vi "Regular Waves (Modded by Matt).vi"(0 "Run":bool, 1 "Wave Period":dbl(slide)=1.0 min=0.5 max=5.0 step=0.01 scale=0.5..5.0 scale format="%.1f", 2 "Wave Height":dbl(slide)=0.1 min=0.0 step=0.001 scale=0.0..0.15606733627984637 scale format="%.3f") -> ()   [LabVIEW 2012]
uses:
  <vilib>/Daq/Ai.llb/AI Read (scaled array).vi
  <vilib>/Daq/ao.llb/AO Write (scaled array).vi
  <vilib>/Daq/ao.llb/AO Write One Update (scaled array).vi
  <vilib>/Analysis/NI_AALBase.lvlib
  <vilib>/Analysis/1siggen.llb/Ramp Pattern by Samples.vi
panel:
  out "Waveform Chart":dbl[][](graph)
  in  "Measure Waves":bool
  in  "Settings":bool
  in  "Power":bool
  out "Buffer Size":i32=4000
  # "Regular Wave Generator"
  # "s"
  # "m"
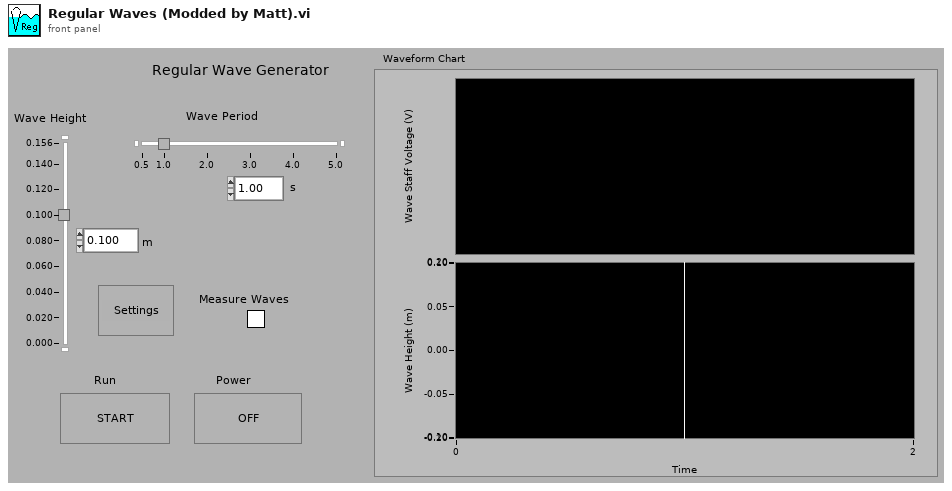
[diagram p1: front panel]
types:
  T1 = cluster{"Output Device":i16, "Output Channel":string, "Sampling Rate (Hz)":dbl, "Input Device":i16, "Input Channel":string, "Input Offset (V)":dbl, "Input Calibration (m/V)":dbl, "Stroke Calibration (V/m)":dbl, "Paddle Height (m)":dbl, "Water Depth (m)":dbl, "Min Period":dbl, "Max Period":dbl, "Max 1/2 Piston Stroke":dbl, "Max H/L":dbl, "Max H/d":dbl}
  T2 = cluster{"Period":dbl, "Wave Height":dbl, "Phase Angle (rad)":dbl}
  T3 = cluster{"Sampling Rate":i32, "Water Depth":dbl, "Paddle Height":dbl}
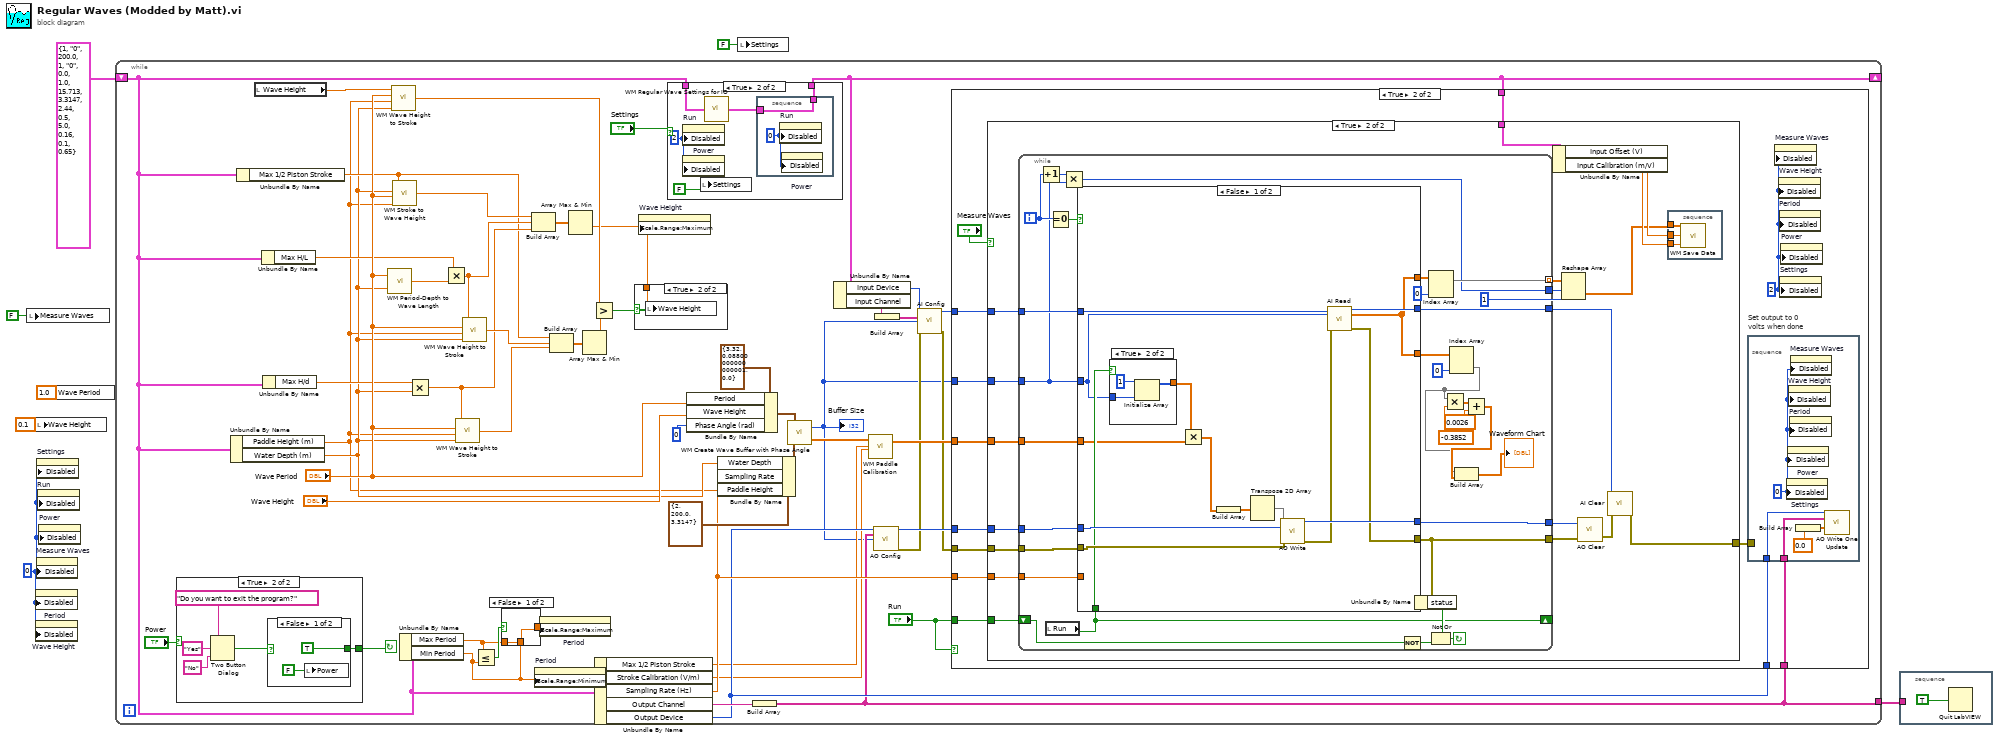
[diagram p0: block diagram]
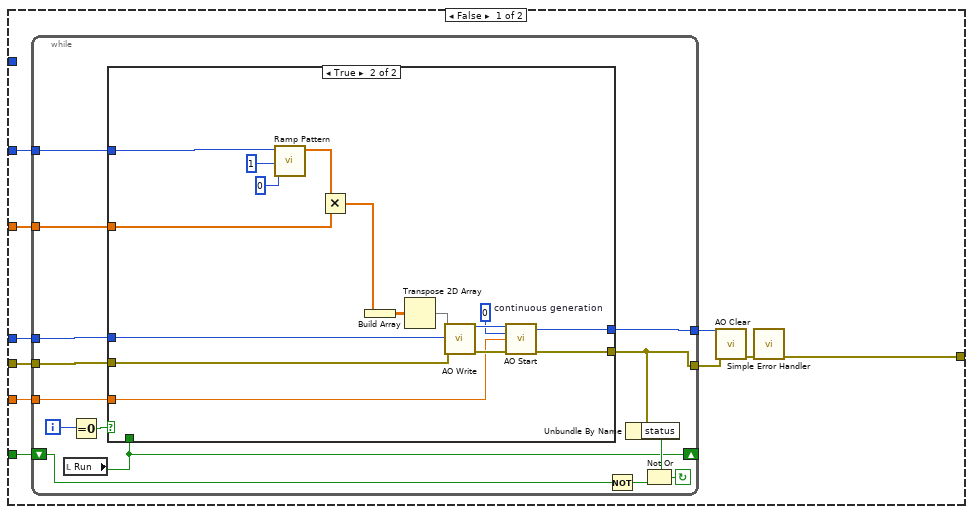
[diagram p3: hidden frame]
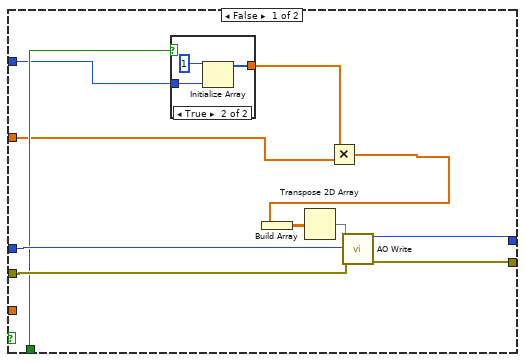
[diagram p4: hidden frame]
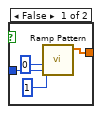
[diagram p5: hidden frame]
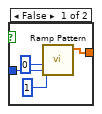
[diagram p6: hidden frame]
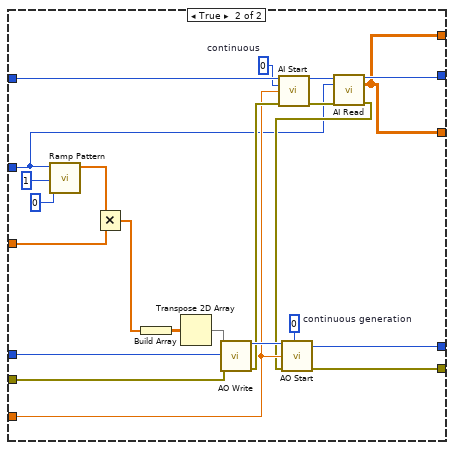
[diagram p7: hidden frame]
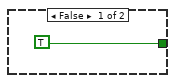
[diagram p9: hidden frame]
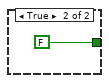
[diagram p10: hidden frame]
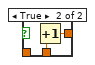
[diagram p11: hidden frame]
diagram:
  w2 = u8 0 ("Write Attribute")
  n1 = local write "Measure Waves"(FALSE ("Measure Waves")) -> ()
  n2 = local write "Wave Height"(0.1 ("Wave Height")) -> ()
  n3 = property on="Period" class="Slide (strict)"("Disabled"=w2) -> ()  [unwired: 2 in, 2 out]
  n4 = property on="Wave Height" class="Slide (strict)"("Disabled"=w2) -> ()  [unwired: 2 in, 2 out]
  n5 = property on="Measure Waves" class="Bool (strict)"("Disabled"=w2) -> ()  [unwired: 2 in, 2 out]
  n6 = property on="Settings" class="Bool (strict)"("Disabled"=w2) -> ()  [unwired: 2 in, 2 out]
  n7 = property on="Run" class="Bool (strict)"("Disabled"=w2) -> ()  [unwired: 2 in, 2 out]
  n8 = property on="Power" class="Bool (strict)"("Disabled"=w2) -> ()  [unwired: 2 in, 2 out]
  n9 = local write "Wave Period"(1.0 ("Period")) -> ()
  n10 = while {
    shift-left: T1 {"Output Device"=1, "Output Channel"="0", "Sampling Rate (Hz)"=200.0, "Input Device"=1, "Input Channel"="0", "Input Offset (V)"=0.0, "Input Calibration (m/V)"=1.0, "Stroke Calibration (V/m)"=15.713, "Paddle Height (m)"=3.3147, "Water Depth (m)"=2.44, "Min Period"=0.5, "Max Period"=5.0, "Max 1/2 Piston Stroke"=0.16, "Max H/L"=0.1, "Max H/d"=0.65} ("Settings") -> [w19]
    shift-right: [w8] -> _
    tunnel: [w27] -> w7
    stop <- w43 continue-if-true
    n11 = case shown="True" "Power" {
      tunnel: [TRUE w240] -> w43
      frame False {
      }
      frame True {
        n12 = Two Button Dialog(message="Do you want to exit the program?", 1:"No" ("F button name (\"Cancel\")"), 2:"Yes" ("T button name (\"OK\")")) -> (T button?=w241:bool)
        n13 = case shown="False" w241 {
          tunnel: [TRUE FALSE] -> w240
          frame False {
            n14 = local write "Power"(FALSE ("Power")) -> ()
          }
          frame True {
          }
        }
      }
    }
    n15 = Unbundle By Name(w19) -> ("Paddle Height (m)"=w22:dbl, "Water Depth (m)"=w23:dbl)
    n16 = Unbundle By Name(w19) -> ("Max 1/2 Piston Stroke"=w26:dbl)
    n17 = local read "Wave Height"() -> (w46:dbl)
    n18 = Unbundle By Name(w19) -> ("Max H/L"=w25:dbl)
    n19 = Unbundle By Name(w19) -> ("Max H/d"=w24:dbl)
    n20 = call "WM Period-Depth to Wave Length.vi"("Water Depth"=w23, "Period"="Wave Period") -> ("WaveLength"=w34:dbl)
    n21 = call "WM Wave Height to Stroke.vi"("Water Depth (m)"=w23, "Flap Height (m)"=w22, "Wave Period (s)"="Wave Period", "Wave Height (m)"=w46) -> ("Flap Amplitude (from x=0) (m)"=w55:dbl)
    n22 = call "WM Stroke to Wave Height.vi"("Paddle Height (m)"=w22, "Wave Period (s)"="Wave Period", "Water Depth (m)"=w23, "Flap Amplitude from x=0 (m)"=w26) -> ("Wave Height (m)"=w50:dbl)
    n23 = Unbundle By Name(w19) -> ("Max Period"=w18:dbl, "Min Period"=w17:dbl)
    n24 = Multiply(x=w24, y=w23) -> (x*y=w33:dbl)
    n25 = Multiply(x=w25, y=w34) -> (x*y=w51:dbl)
    n26 = call "WM Wave Height to Stroke.vi"("Water Depth (m)"=w23, "Flap Height (m)"=w22, "Wave Period (s)"="Wave Period", "Wave Height (m)"=w33) -> ("Flap Amplitude (from x=0) (m)"=w49:dbl)
    n27 = call "WM Wave Height to Stroke.vi"("Water Depth (m)"=w23, "Flap Height (m)"=w22, "Wave Period (s)"="Wave Period", "Wave Height (m)"=w51) -> ("Flap Amplitude (from x=0) (m)"=w48:dbl)
    n28 = Less Or Equal?(x=w18, y=w17) -> (x <= y?=w56:bool)
    n29 = case shown="False" w56 {
      tunnel: w17 -> [_ w250]
      tunnel: [w248 w249] -> w45
      tunnel: w18 -> [w248 _]
      frame False {
      }
      frame True {
        n30 = Increment(x=w250) -> (x+1=w249:dbl)
      }
    }
    n31 = Build Array(w50, w51, w33) -> (w54:dbl[])
    n32 = property on="Period" class="Slide (strict)"("Scale.Range:Minimum"=w17) -> ()  [unwired: 2 in, 2 out]
    n33 = property on="Period" class="Slide (strict)"("Scale.Range:Maximum"=w45) -> ()  [unwired: 2 in, 2 out]
    n34 = Build Array(w26, w48, w49) -> (w53:dbl[])
    n35 = Array Max & Min(array=w54) -> (min value=w47:dbl)  [unwired: 3 out]
    n36 = Array Max & Min(array=w53) -> (min value=w52:dbl)  [unwired: 3 out]
    n37 = Greater?(x=w55, y=w52) -> (0:w57:bool)
    n38 = Unbundle By Name(w19) -> ("Max 1/2 Piston Stroke"=w21:dbl, "Stroke Calibration (V/m)"=w20:dbl, "Sampling Rate (Hz)"=w30:dbl, "Output Channel"=w29:string, "Output Device"=w28:i16)
    n39 = case shown="True" w57 {
      tunnel: w47 -> [_ w251]
      frame False {
      }
      frame True {
        n40 = local write "Wave Height"(w251) -> ()
      }
    }
    n41 = property on="Wave Height" class="Slide (strict)"("Scale.Range:Maximum"=w47) -> ()  [unwired: 2 in, 2 out]
    n42 = case shown="True" "Settings" {
      tunnel: w19 -> [w231 w236]
      tunnel: [w231 w234] -> w8
      frame False {
      }
      frame True {
        w232 = u8 2 ("Write Attribute")
        n43 = property on="Run" class="Bool (strict)"("Disabled"=w232) -> ()  [unwired: 2 in, 2 out]
        n44 = property on="Power" class="Bool (strict)"("Disabled"=w232) -> ()  [unwired: 2 in, 2 out]
        n45 = local write "Settings"(FALSE ("Settings")) -> ()
        n46 = call "WM Regular Wave Settings for IO.vi"("Settings"=w236) -> ("Settings Output"=w235:T1)
        n47 = stacked-sequence {
          tunnel: w235 -> [w238]
          tunnel: [w238] -> w234
          frame #0 {
            w237 = u8 0 ("Write Attribute")
            n48 = property on="Run" class="Bool (strict)"("Disabled"=w237) -> ()  [unwired: 2 in, 2 out]
            n49 = property on="Power" class="Bool (strict)"("Disabled"=w237) -> ()  [unwired: 2 in, 2 out]
          }
        }
      }
    }
    n50 = Bundle By Name(cluster=T2 {"Period"=3.32, "Wave Height"=0.08800000000000001, "Phase Angle (rad)"=0.0} ("Sine Paramaters"), "Period"="Wave Period", "Wave Height"="Wave Height", "Phase Angle (rad)"=0) -> (w37:T2)
    n51 = Bundle By Name(cluster=T3 {"Sampling Rate"=2, "Water Depth"=200.0, "Paddle Height"=3.3147} ("Buffer Info"), "Water Depth"=w23, "Sampling Rate"=w30, "Paddle Height"=w22) -> (w39:T3)
    n52 = Build Array(w29) -> (w27:string[])
    n53 = call "WM Create Wave Buffer with Phase Angle.vi"("Buffer Info"=w39, "Sine Paramaters"=w37) -> ("Output"=w42:dbl[], "Buffer Size"=w11:i32)
    "Buffer Size" <- w11
    n54 = Unbundle By Name(w8) -> ("Input Device"=w12:i16, "Input Channel"=w14:string)
    n55 = call "WM Paddle Calibration.vi"("Stroke Calibration (V/m)"=w20, "Max 1/2 Piston Stroke (m)"=w21, "Input Stroke Distance (m)"=w42) -> ("Output Voltage"=w41:dbl[])  [unwired: 1 in, 1 out]
    n56 = call <vilib>:"AO Config.vi"("device (1)"=w28, "channels (0)"=w27, "buffer size (1000 updates)"=w11) -> ("taskID"=w58:u32, "error out"=w16:errorcluster)  [unwired: 10 in, 1 out]
    n57 = Build Array(w14) -> (w13:string[])
    n58 = call <vilib>:"AI Config.vi"("device (1)"=w12, "channels (0)"=w13, "buffer size (1000 scans)"=w11, "error in (no error)"=w16) -> ("taskID"=w10:u32, "error out"=w15:errorcluster)  [unwired: 9 in, 1 out]
    n59 = case shown="True" "Run" {
      tunnel: w15 -> [_ w71]
      tunnel: w58 -> [_ w70]
      tunnel: w27 -> [_ w68]
      tunnel: w11 -> [_ w67]
      tunnel: "Run" -> [_ w66]
      tunnel: w41 -> [_ w65]
      tunnel: w30 -> [_ w64]
      tunnel: w28 -> [_ w63]
      tunnel: w10 -> [_ w62]
      tunnel: w8 -> [_ w59]
      frame False {
      }
      frame True {
        w60 = u8 2 ("Write Attribute")
        n60 = case shown="True" "Measure Waves" {
          tunnel: w71 -> [w73 w142]
          tunnel: w70 -> [w81 w146]
          tunnel: [w79 w137] -> w69
          tunnel: w67 -> [w77 w148]
          tunnel: w66 -> [w76 w145]
          tunnel: w65 -> [w75 w147]
          tunnel: w64 -> [w74 w144]
          tunnel: w62 -> [_ w143]
          tunnel: w59 -> [_ w136]
          frame False {
            n61 = while {
              tunnel: [w83] -> w72
              tunnel: w73 -> [w84]
              tunnel: w77 -> [w85]
              tunnel: w75 -> [w86]
              tunnel: w74 -> [w87]
              shift-left: w76 -> [w88]
              shift-right: [w82] -> _
              tunnel: [w92] -> w78
              tunnel: w81 -> [w93]
              i -> [w95]
              stop <- w89 continue-if-true
              n62 = local read "Run"() -> (w82:bool)
              n63 = Equal To 0?(x=w95) -> (x = 0?=w94:bool)
              n64 = case shown="True" w94 {
                tunnel: w93 -> [w106 w124]
                tunnel: w84 -> [w105 w123]
                tunnel: [w104 w125] -> w92
                tunnel: [w103 w122] -> w83
                tunnel: w87 -> [_ w121]
                tunnel: w82 -> [w101 _]
                tunnel: w86 -> [w98 w115]
                tunnel: w85 -> [w97 w116]
                frame False {
                  n65 = case shown="True" w101 {
                    tunnel: [w110 w111] -> w102
                    tunnel: w97 -> [w107 w113]
                    frame False {
                      n66 = call-poly <vilib>:"Ramp Pattern.vi"("start"=1, "end"=0, "samples"=w107) -> ("Ramp Pattern"=w110:dbl[])  [unwired: 7 in, 1 out]
                    }
                    frame True {
                      n67 = Initialize Array(1, w113) -> (w111:i32[])
                    }
                  }
                  n68 = Multiply(x=w102, y=w98) -> (x*y=w96:dbl[])
                  n69 = Build Array(w96) -> (w100:dbl[][])
                  n70 = Transpose 2D Array(2D array=w100) -> (transposed array=w99:dbl[][])
                  n71 = call-poly <vilib>:"AO Write.vi"("taskID in"=w106, "scaled data"=w99, "error in (no error)"=w105) -> ("taskID out"=w104:u32, "error out"=w103:errorcluster)  [unwired: 8 in, 3 out]
                }
                frame True {
                  w126 = 0  # continuous generation
                  n72 = call-poly <vilib>:"Ramp Pattern.vi"("start"=0, "end"=1, "samples"=w116) -> ("Ramp Pattern"=w118:dbl[])  [unwired: 7 in, 1 out]
                  n73 = Multiply(x=w118, y=w115) -> (x*y=w114:dbl[])
                  n74 = Build Array(w114) -> (w129:dbl[][])
                  n75 = Transpose 2D Array(2D array=w129) -> (transposed array=w117:dbl[][])
                  n76 = call-poly <vilib>:"AO Write.vi"("taskID in"=w124, "scaled data"=w117, "error in (no error)"=w123) -> ("taskID out"=w127:u32, "error out"=w128:errorcluster)  [unwired: 8 in, 3 out]
                  n77 = call <vilib>:"AO Start.vi"("taskID in"=w127, "number of buffer iterations (1)"=w126, "update rate (1000 updates/sec)"=w121, "error in (no error)"=w128) -> ("taskID out"=w125:u32, "error out"=w122:errorcluster)  [unwired: 9 in, 1 out]
                }
              }
              n78 = Not(x=w88) -> (.not. x?=w90:bool)
              n79 = Unbundle By Name(w83) -> ("status"=w91:bool)
              n80 = Not Or(1:w90, 2:w91) -> (0:w89:bool)
            }
            n81 = call <vilib>:"AO Clear.vi"("error in (no error)"=w72, "taskID in"=w78) -> ("error out"=w80:errorcluster)  [unwired: 4 in, 1 out]
            n82 = call <vilib>:"Simple Error Handler.vi"("error in (no error)"=w80) -> ("error out"=w79:errorcluster)  [unwired: 4 in, 4 out]
          }
          frame True {
            n83 = while {
              tunnel: [w158] -> w131
              tunnel: [w163] -> w133 mode=indexing
              tunnel: [w165] -> w141
              tunnel: w142 -> [w166]
              tunnel: [w157] -> w139
              tunnel: w143 -> [w167]
              tunnel: w148 -> [w159]
              tunnel: w147 -> [w169]
              tunnel: w144 -> [w170]
              shift-left: w145 -> [w171]
              shift-right: [w168] -> _
              tunnel: [w175] -> w140
              tunnel: w146 -> [w176]
              i -> [w161]
              stop <- w172 continue-if-true
              n84 = Increment(x=w161) -> (x+1=w160:i32)
              n85 = local read "Run"() -> (w168:bool)
              n86 = Equal To 0?(x=w161) -> (x = 0?=w177:bool)
              n87 = Multiply(x=w160, y=w159) -> (x*y=w158:i32)
              n88 = case shown="False" w177 {
                tunnel: w176 -> [w192 w218]
                tunnel: w166 -> [w191 w217]
                tunnel: [w190 w219] -> w175
                tunnel: [w179 w216] -> w165
                tunnel: w170 -> [_ w207]
                tunnel: w168 -> [w188 _]
                tunnel: w169 -> [w185 w211]
                tunnel: w159 -> [w181 w201]
                tunnel: w167 -> [w182 w208]
                tunnel: [w180 w202] -> w157
                tunnel: [w178 w200] -> w164
                tunnel: [w178 w200] -> w152
                frame False {
                  n89 = case shown="True" w188 {
                    tunnel: [w196 w197] -> w189
                    tunnel: w181 -> [w193 w199]
                    frame False {
                      n90 = call-poly <vilib>:"Ramp Pattern.vi"("start"=1, "end"=0, "samples"=w193) -> ("Ramp Pattern"=w196:dbl[])  [unwired: 7 in, 1 out]
                    }
                    frame True {
                      n91 = Initialize Array(1, w199) -> (w197:i32[])
                    }
                  }
                  n92 = Multiply(x=w189, y=w185) -> (x*y=w184:dbl[])
                  n93 = Build Array(w184) -> (w187:dbl[][])
                  n94 = Transpose 2D Array(2D array=w187) -> (transposed array=w186:dbl[][])
                  n95 = call-poly <vilib>:"AO Write.vi"("taskID in"=w192, "scaled data"=w186, "error in (no error)"=w191) -> ("taskID out"=w190:u32, "error out"=w183:errorcluster)  [unwired: 8 in, 3 out]
                  n96 = call-poly <vilib>:"AI Read.vi"("taskID in"=w182, "number of scans to read (-1:all)"=w181, "error in (no error)"=w183) -> ("taskID out"=w180:u32, "scaled data"=w178:sgl[][], "error out"=w179:errorcluster)  [unwired: 7 in, 3 out]
                }
                frame True {
                  w206 = 0  # continuous
                  w220 = 0  # continuous generation
                  n97 = call-poly <vilib>:"Ramp Pattern.vi"("start"=0, "end"=1, "samples"=w201) -> ("Ramp Pattern"=w213:dbl[])  [unwired: 7 in, 1 out]
                  n98 = Multiply(x=w213, y=w211) -> (x*y=w210:dbl[])
                  n99 = Build Array(w210) -> (w222:dbl[][])
                  n100 = Transpose 2D Array(2D array=w222) -> (transposed array=w212:dbl[][])
                  n101 = call-poly <vilib>:"AO Write.vi"("taskID in"=w218, "scaled data"=w212, "error in (no error)"=w217) -> ("taskID out"=w221:u32, "error out"=w209:errorcluster)  [unwired: 8 in, 3 out]
                  n102 = call <vilib>:"AI Start.vi"("taskID in"=w208, "number of scans to acquire (-1)"=w206, "scan rate (1000 scans/sec)"=w207, "error in (no error)"=w209) -> ("taskID out"=w205:u32, "error out"=w204:errorcluster)  [unwired: 8 in, 2 out]
                  n103 = call-poly <vilib>:"AI Read.vi"("taskID in"=w205, "number of scans to read (-1:all)"=w201, "error in (no error)"=w204) -> ("taskID out"=w202:u32, "scaled data"=w200:sgl[][], "error out"=w203:errorcluster)  [unwired: 7 in, 3 out]
                  n104 = call <vilib>:"AO Start.vi"("taskID in"=w221, "number of buffer iterations (1)"=w220, "update rate (1000 updates/sec)"=w207, "error in (no error)"=w203) -> ("taskID out"=w219:u32, "error out"=w216:errorcluster)  [unwired: 9 in, 1 out]
                }
              }
              n105 = Not(x=w171) -> (.not. x?=w173:bool)
              n106 = Unbundle By Name(w165) -> ("status"=w174:bool)
              n107 = Index Array(array=w164, index (col)=0 ("Index")) -> (element=w163:sgl[])  [unwired: 1 in]
              n108 = Not Or(1:w173, 2:w174) -> (0:w172:bool)
              n109 = Index Array(array=w152, index (col)=0 ("disabled index (col)")) -> (element=w150:sgl[])  [unwired: 1 in]
              n110 = Multiply(x=w150, y=-0.3852) -> (x*y=w155:dbl[])
              n111 = Add(x=w155, y=0.0026) -> (x+y=w151:dbl[])
              n112 = Build Array(w150, w151) -> (→"Waveform Chart":dbl[][])
            }
            n113 = Unbundle By Name(w136) -> ("Input Offset (V)"=w135:dbl, "Input Calibration (m/V)"=w134:dbl)
            n114 = Reshape Array(w133, w131, 1 ("Dimension Size")) -> (w132:sgl[][])
            n115 = call <vilib>:"AO Clear.vi"("error in (no error)"=w141, "taskID in"=w140) -> ("error out"=w138:errorcluster)  [unwired: 4 in, 1 out]
            n116 = call <vilib>:"AI Clear.vi"("error in (no error)"=w138, "taskID in"=w139) -> ("error out"=w137:errorcluster)  [unwired: 4 in, 1 out]
            n117 = stacked-sequence {
              tunnel: w132 -> [w225]
              tunnel: w135 -> [w224]
              tunnel: w134 -> [w223]
              frame #0 {
                n118 = call "WM Save Data.vi"("Input Calibration"=w223, "Input Offset"=w224, "Input Data"=w225) -> ()
              }
            }
          }
        }
        n119 = stacked-sequence "Set output to 0\nvolts when done" {
          tunnel: w69 -> [_]
          tunnel: w63 -> [w228]
          tunnel: w68 -> [w227]
          frame #0 {
            w226 = u8 0 ("Write Attribute")
            n120 = property on="Settings" class="Bool (strict)"("Disabled"=w226) -> ()  [unwired: 2 in, 2 out]
            n121 = property on="Power" class="Bool (strict)"("Disabled"=w226) -> ()  [unwired: 2 in, 2 out]
            n122 = property on="Wave Height" class="Slide (strict)"("Disabled"=w226) -> ()  [unwired: 2 in, 2 out]
            n123 = property on="Period" class="Slide (strict)"("Disabled"=w226) -> ()  [unwired: 2 in, 2 out]
            n124 = property on="Measure Waves" class="Bool (strict)"("Disabled"=w226) -> ()  [unwired: 2 in, 2 out]
            n125 = Build Array(sgl 0.0 ("Set analog output to 0")) -> (w230:sgl[])
            n126 = call-poly <vilib>:"AO Write One Update.vi"("device (1)"=w228, "channels (0)"=w227, "scaled data"=w230) -> ()  [unwired: 12 in, 1 out]
          }
        }
        n127 = property on="Measure Waves" class="Bool (strict)"("Disabled"=w60) -> ()  [unwired: 2 in, 2 out]
        n128 = property on="Wave Height" class="Slide (strict)"("Disabled"=w60) -> ()  [unwired: 2 in, 2 out]
        n129 = property on="Period" class="Slide (strict)"("Disabled"=w60) -> ()  [unwired: 2 in, 2 out]
        n130 = property on="Settings" class="Bool (strict)"("Disabled"=w60) -> ()  [unwired: 2 in, 2 out]
        n131 = property on="Power" class="Bool (strict)"("Disabled"=w60) -> ()  [unwired: 2 in, 2 out]
      }
    }
  }
  n132 = local write "Settings"(FALSE ("Settings")) -> ()
  n133 = stacked-sequence {
    tunnel: w7 -> [_]
    frame #0 {
      n134 = Quit LabVIEW(quit? (T)=TRUE) -> ()
    }
  }
